vi "CRYStepSetup.vi"() -> ()   [LabVIEW 2013]
uses:
  CRYStepSetup Global.vi
panel:
  in  "StateOut":bool
  in  "Add Graph":bool
  in  "IconRing":u16(ring)
  in  "Add Graph Menu":bool
  in  "Control Visible":bool
  in  "Property":bool
  in  "TitleShowOnOff":bool
  in  "Save As":bool
  in  "Load":bool
  in  "Revert":bool
  out "SubVI Ref":refnum<vi>
  in  "stop":bool
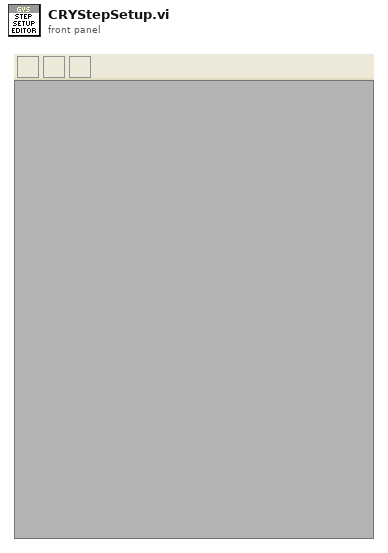
[diagram p1: front panel]
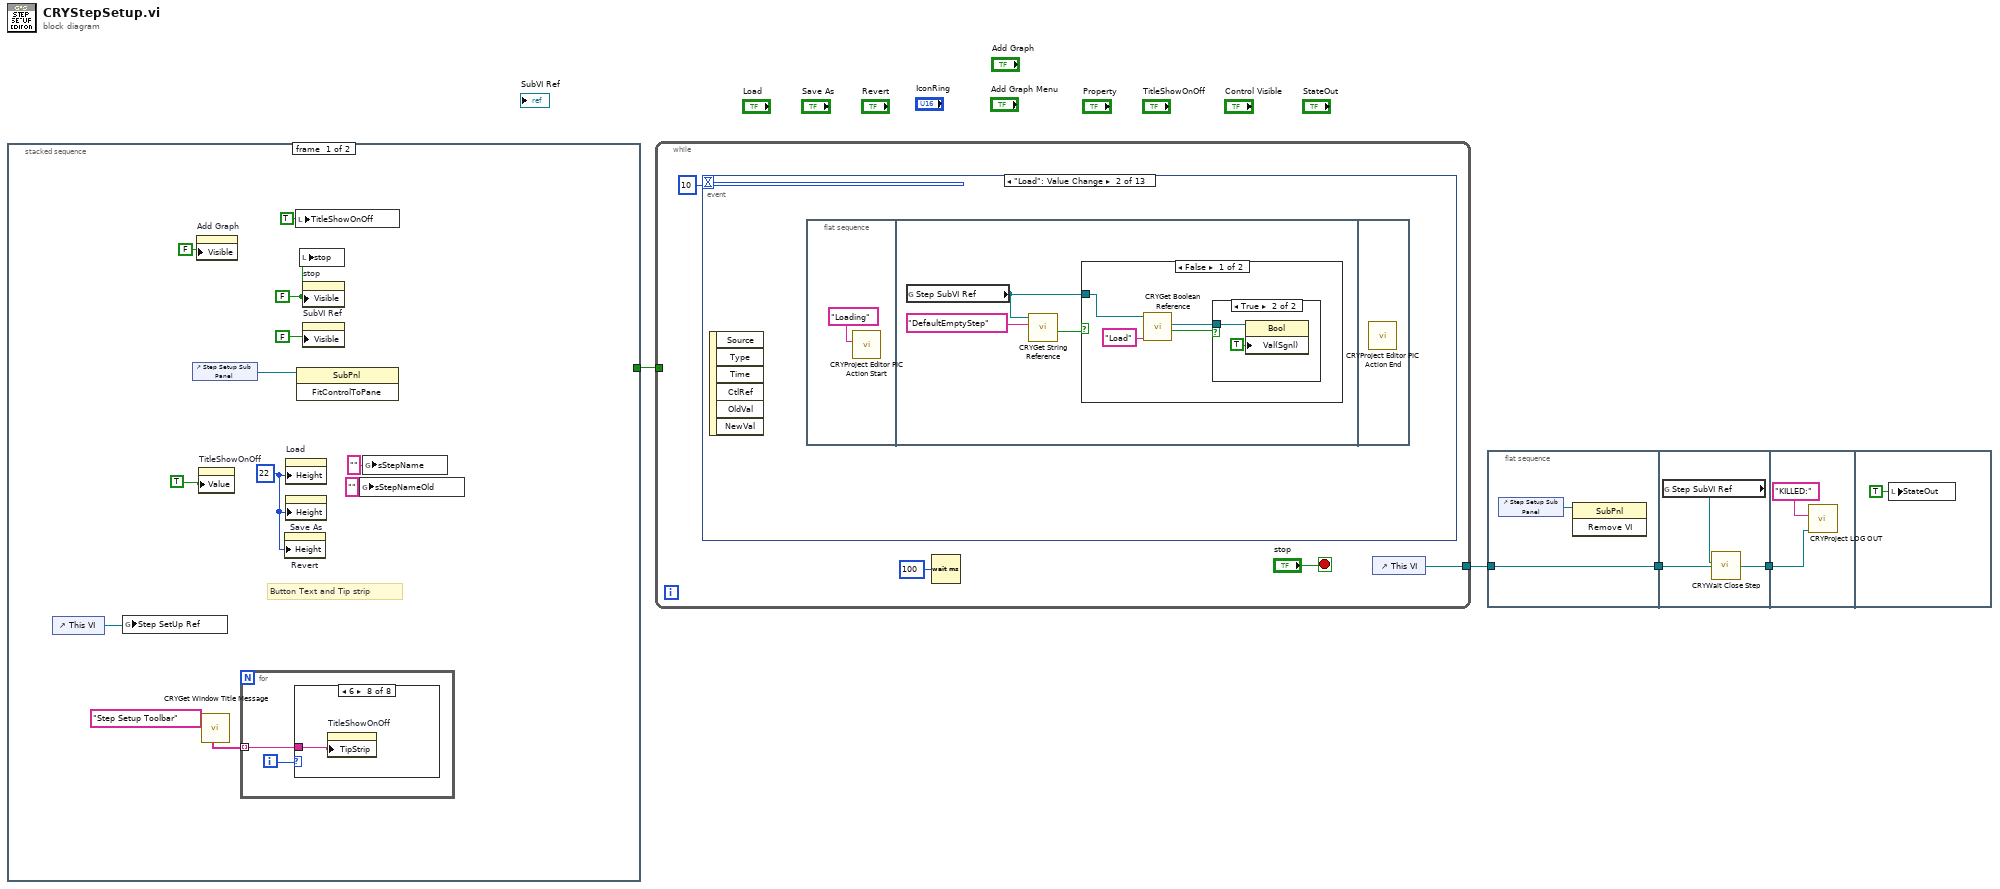
[diagram p0: block diagram]
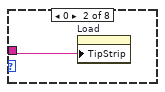
[diagram p3: hidden frame]
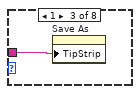
[diagram p4: hidden frame]
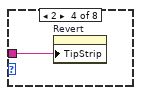
[diagram p5: hidden frame]
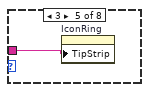
[diagram p6: hidden frame]
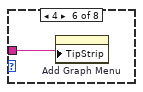
[diagram p7: hidden frame]
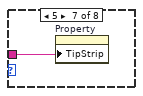
[diagram p8: hidden frame]
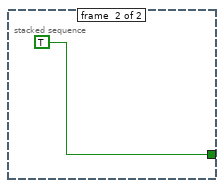
[diagram p9: hidden frame]
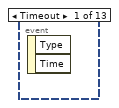
[diagram p10: hidden frame]
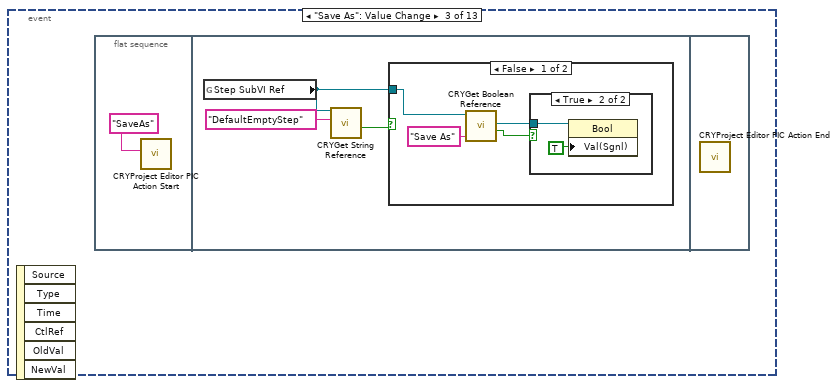
[diagram p13: hidden frame]
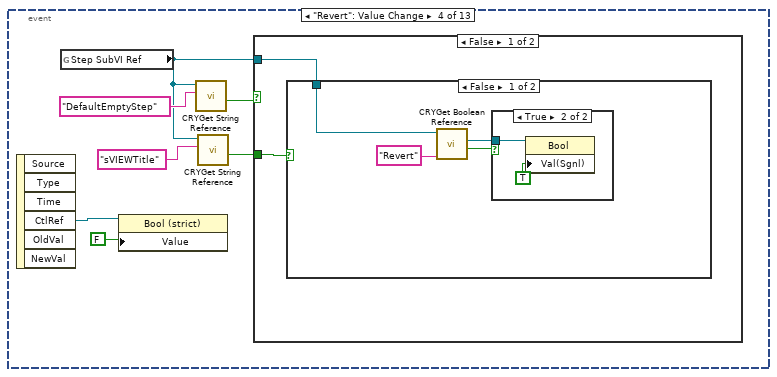
[diagram p16: hidden frame]
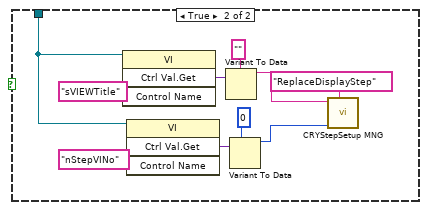
[diagram p18: hidden frame]
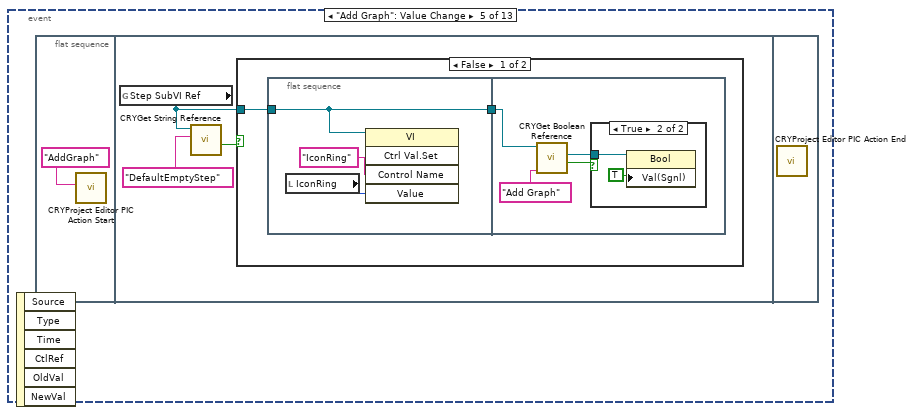
[diagram p20: hidden frame]
diagram:
  n1 = stacked-sequence {
    tunnel: [_ TRUE ("Step Setup Exist")] -> w4
    frame #0 {
      w15 = u32 22 ("Button Size:Height")
      w13 = FALSE ("Visible")
      # "Button Text and Tip strip"
      n2 = control-ref of="This VI"() -> (w5:refnum<vi>)
      n3 = global write "CRYStepSetup Global.vi" "Step SetUp Ref"(w5) -> ()
      n4 = control-ref of="Step Setup Sub Panel"() -> (w9:refnum<vi>)
      n5 = property on="Add Graph" class="Bool (strict)"("Visible"=FALSE) -> ()  [unwired: 2 in, 2 out]
      n6 = property on="TitleShowOnOff" class="Bool (strict)"("Value"=TRUE ("TitleShowOnOff")) -> ()  [unwired: 2 in, 2 out]
      n7 = call "CRYGet Window Title Message.vi"("Kind"="Step Setup Toolbar") -> ("Tip Strip"=w6:string[])  [unwired: 5 in, 5 out]
      n8 = for {
        tunnel: w6 -> [w17] mode=indexing
        i -> [w18]
        n9 = case shown="6" w18 {
          tunnel: w17 -> [_ w19 w20 w21 w22 w23 w24 w25]
          frame Default {
          }
          frame 0 {
            n10 = property on="Load" class="Bool (strict)"("TipStrip"=w19) -> ()  [unwired: 2 in, 2 out]
          }
          frame 1 {
            n11 = property on="Save As" class="Bool (strict)"("TipStrip"=w20) -> ()  [unwired: 2 in, 2 out]
          }
          frame 2 {
            n12 = property on="Revert" class="Bool (strict)"("TipStrip"=w21) -> ()  [unwired: 2 in, 2 out]
          }
          frame 3 {
            n13 = property on="IconRing" class="Ring (strict)"("TipStrip"=w22) -> ()  [unwired: 2 in, 2 out]
          }
          frame 4 {
            n14 = property on="Add Graph Menu" class="Bool (strict)"("TipStrip"=w23) -> ()  [unwired: 2 in, 2 out]
          }
          frame 5 {
            n15 = property on="Property" class="Bool (strict)"("TipStrip"=w24) -> ()  [unwired: 2 in, 2 out]
          }
          frame 6 {
            n16 = property on="TitleShowOnOff" class="Bool (strict)"("TipStrip"=w25) -> ()  [unwired: 2 in, 2 out]
          }
        }
      }
      n17 = property on="Revert" class="Bool (strict)"("Height"=w15) -> ()  [unwired: 2 in, 2 out]
      n18 = property on="Load" class="Bool (strict)"("Height"=w15) -> ()  [unwired: 2 in, 2 out]
      n19 = property on="Save As" class="Bool (strict)"("Height"=w15) -> ()  [unwired: 2 in, 2 out]
      n20 = local write "TitleShowOnOff"(TRUE ("TitleShowOnOff")) -> ()
      n21 = invoke class="SubPnl" method="FitControlToPane"(reference=w9) -> ()  [unwired: 2 in, 3 out]
      n22 = local write "stop"(w13) -> ()
      n23 = property on="stop" class="Bool (strict)"("Visible"=w13) -> ()  [unwired: 2 in, 2 out]
      n24 = property on="SubVI Ref" class="VIRef (strict)"("Visible"=FALSE) -> ()  [unwired: 2 in, 2 out]
      n25 = global write "CRYStepSetup Global.vi" "sStepNameOld"("" ("sStepName")) -> ()
      n26 = global write "CRYStepSetup Global.vi" "sStepName"("" ("sStepName")) -> ()
    }
    frame #1 {
    }
  }
  n27 = while {
    tunnel: w4 -> [_]
    tunnel: [w29] -> w3
    stop <- "stop" stop-if-true
    n28 = event shown="[1] \"Load\": Value Change" {
      selector: _ -> [_ _ _ _ _ _ _ _ _ _ _ _ _]
      dyn-events: _ -> [_ _ _ _ _ _ _ _ _ _ _ _ _]
      timeout: 10 -> [_ _ _ _ _ _ _ _ _ _ _ _ _]
      event Timeout {
        n29 = event-data() -> ()  [unwired: 3 out]
      }
      event "Load": Value Change {
        n30 = event-data() -> ()  [unwired: 7 out]
        n31 = flat-sequence {
          frame #0 {
            n32 = call "CRYProject Editor PIC Action Start.vi"("sData"="Loading" ("StateLabel")) -> ()  [unwired: 11 in]
          }
          frame #1 {
            n33 = global read "CRYStepSetup Global.vi" "Step SubVI Ref"() -> (w32:refnum<vi>)
            n34 = call "CRYGet String Reference.vi"("Label Name"="DefaultEmptyStep" ("element"), "VI Refnum"=w32) -> ("Find?"=w33:bool)  [unwired: 9 out]
            n35 = case shown="False" w33 {
              tunnel: w32 -> [w36 _]
              frame False {
                n36 = call "CRYGet Boolean Reference.vi"("Label Name"="Load", "VI Refnum"=w36) -> ("Exist?"=w35:bool, "Boolean Ref"=w38:refnum<vi>)  [unwired: 8 out]
                n37 = case shown="True" w35 {
                  tunnel: w38 -> [_ w40]
                  frame False {
                  }
                  frame True {
                    n38 = property class="Bool"(reference=w40, "Val(Sgnl)"=TRUE ("Value")) -> ()  [unwired: 1 in, 2 out]
                  }
                }
              }
              frame True {
              }
            }
          }
          frame #2 {
            n39 = call "CRYProject Editor PIC Action End.vi"() -> ()  [unwired: 12 in]
          }
        }
      }
      event "Save As": Value Change {
        n40 = event-data() -> ()  [unwired: 7 out]
        n41 = flat-sequence {
          frame #0 {
            n42 = call "CRYProject Editor PIC Action Start.vi"("sData"="SaveAs" ("StateLabel")) -> ()  [unwired: 11 in]
          }
          frame #1 {
            n43 = global read "CRYStepSetup Global.vi" "Step SubVI Ref"() -> (w42:refnum<vi>)
            n44 = call "CRYGet String Reference.vi"("Label Name"="DefaultEmptyStep" ("element"), "VI Refnum"=w42) -> ("Find?"=w43:bool)  [unwired: 9 out]
            n45 = case shown="False" w43 {
              tunnel: w42 -> [w46 _]
              frame False {
                n46 = call "CRYGet Boolean Reference.vi"("Label Name"="Save As" ("Label.Text"), "VI Refnum"=w46) -> ("Exist?"=w45:bool, "Boolean Ref"=w48:refnum<vi>)  [unwired: 8 out]
                n47 = case shown="True" w45 {
                  tunnel: w48 -> [_ w50]
                  frame False {
                  }
                  frame True {
                    n48 = property class="Bool"(reference=w50, "Val(Sgnl)"=TRUE ("Value")) -> ()  [unwired: 1 in, 2 out]
                  }
                }
              }
              frame True {
              }
            }
          }
          frame #2 {
            n49 = call "CRYProject Editor PIC Action End.vi"() -> ()  [unwired: 12 in]
          }
        }
      }
      event "Revert": Value Change {
        n50 = event-data() -> ("CtlRef"=w57:refnum<vi>)  [unwired: 6 out]
        n51 = global read "CRYStepSetup Global.vi" "Step SubVI Ref"() -> (w53:refnum<vi>)
        n52 = property class="Bool (strict)"(reference=w57, "Value"=FALSE) -> ()  [unwired: 1 in, 2 out]
        n53 = call "CRYGet String Reference.vi"("Label Name"="DefaultEmptyStep" ("element"), "VI Refnum"=w53) -> ("Find?"=w54:bool)  [unwired: 9 out]
        n54 = call "CRYGet String Reference.vi"("Label Name"="sVIEWTitle" ("Control Name"), "VI Refnum"=w53) -> ("Find?"=w51:bool)  [unwired: 9 out]
        n55 = case shown="False" w54 {
          tunnel: w53 -> [w59 _]
          tunnel: w51 -> [w58 _]
          frame False {
            n56 = case shown="False" w58 {
              tunnel: w59 -> [w61 w70]
              frame False {
                n57 = call "CRYGet Boolean Reference.vi"("Label Name"="Revert" ("Label.Text"), "VI Refnum"=w61) -> ("Exist?"=w60:bool, "Boolean Ref"=w63:refnum<vi>)  [unwired: 8 out]
                n58 = case shown="True" w60 {
                  tunnel: w63 -> [_ w65]
                  frame False {
                  }
                  frame True {
                    n59 = property class="Bool"(reference=w65, "Val(Sgnl)"=TRUE ("Value")) -> ()  [unwired: 1 in, 2 out]
                  }
                }
              }
              frame True {
                n60 = invoke class="VI" method="Ctrl Val.Get"(reference=w70, "Control Name"="sVIEWTitle") -> ("Get Control Value Variant"=w74:variant)  [unwired: 2 in, 3 out]
                n61 = invoke class="VI" method="Ctrl Val.Get"(reference=w70, "Control Name"="nStepVINo") -> ("Get Control Value Variant"=w71:variant)  [unwired: 2 in, 3 out]
                n62 = Variant To Data(type="", Variant=w74) -> (data=w73:string)  [unwired: 1 in, 1 out]
                n63 = Variant To Data(type=0, Variant=w71) -> (data=w69:i32)  [unwired: 1 in, 1 out]
                n64 = call "CRYStepSetup MNG.vi"("sAction"="ReplaceDisplayStep", "nData"=w69, "sData"=w73) -> ()  [unwired: 7 in, 2 out]
              }
            }
          }
          frame True {
          }
        }
      }
      event "Add Graph": Value Change {
        n65 = event-data() -> ()  [unwired: 7 out]
        n66 = flat-sequence {
          frame #0 {
            n67 = call "CRYProject Editor PIC Action Start.vi"("sData"="AddGraph" ("StateLabel")) -> ()  [unwired: 11 in]
          }
          frame #1 {
            n68 = global read "CRYStepSetup Global.vi" "Step SubVI Ref"() -> (w77:refnum<vi>)
            n69 = call "CRYGet String Reference.vi"("Label Name"="DefaultEmptyStep" ("element"), "VI Refnum"=w77) -> ("Find?"=w78:bool)  [unwired: 9 out]
            n70 = case shown="False" w78 {
              tunnel: w77 -> [w80 _]
              frame False {
                n71 = flat-sequence {
                  tunnel: [w84] -> w81
                  tunnel: w80 -> [w84]
                  tunnel: w81 -> [w86]
                  frame #0 {
                    n72 = local read "IconRing"() -> (w83:u16)
                    n73 = invoke class="VI" method="Ctrl Val.Set"(reference=w84, "Control Name"="IconRing", "Value"=w83) -> ()  [unwired: 2 in, 5 out]
                  }
                  frame #1 {
                    n74 = call "CRYGet Boolean Reference.vi"("Label Name"="Add Graph" ("Label.Text"), "VI Refnum"=w86) -> ("Exist?"=w85:bool, "Boolean Ref"=w88:refnum<vi>)  [unwired: 8 out]
                    n75 = case shown="True" w85 {
                      tunnel: w88 -> [_ w90]
                      frame False {
                      }
                      frame True {
                        n76 = property class="Bool"(reference=w90, "Val(Sgnl)"=TRUE ("Value")) -> ()  [unwired: 1 in, 2 out]
                      }
                    }
                  }
                }
              }
              frame True {
              }
            }
          }
          frame #2 {
            n77 = call "CRYProject Editor PIC Action End.vi"() -> ()  [unwired: 12 in]
          }
        }
      }
      event "IconRing": Mouse Down? {
        n78 = event-data() -> ()  [unwired: 9 out]
        n79 = flat-sequence {
          frame #0 {
            n80 = call "CRYProject Editor PIC Action Start.vi"("sData"="AddGraph" ("StateLabel")) -> ()  [unwired: 11 in]
          }
          frame #1 {
            n81 = property on="Add Graph" class="Bool (strict)"("Val(Sgnl)"=TRUE ("Value (Signaling)")) -> ()  [unwired: 2 in, 2 out]
          }
          frame #2 {
            n82 = call "CRYProject Editor PIC Action End.vi"() -> ()  [unwired: 12 in]
          }
        }
        n83 = event-data() -> ()  [unwired: 5 in, 1 out]
      }
      event "Add Graph Menu": Mouse Down? {
        n84 = event-data() -> ()  [unwired: 9 out]
        n85 = event-data("Button"=u16 2) -> ()  [unwired: 4 in, 1 out]
      }
      event "Add Graph Menu": Shortcut Menu Activation? {
        w96 = string[] ["Wave Graph", "XY Graph", "Polar", "Table", "Result", "Bar", "Text", "Digital", "Picture", "Intensity"]
        n86 = event-data() -> ("MenuRef"=w94:refnum<k9>)  [unwired: 7 out]
        n87 = Delete Menu Items(9:w94) -> (3:w95:refnum<k9>)  [unwired: 3 in, 1 out]
        n88 = Insert Menu Items(7:w96, 8:w96, 9:w95) -> ()  [unwired: 3 in, 3 out]
        n89 = event-data() -> ()  [unwired: 2 in, 1 out]
      }
      event "Add Graph Menu": Shortcut Menu Selection (User) {
        n90 = event-data() -> ("ItemTag"=w98:string)  [unwired: 8 out]
        n91 = flat-sequence {
          tunnel: [w99] -> _
          tunnel: "Below" ("ItemTag") -> [w103]
          tunnel: w98 -> [w99]
          frame #0 {
            n92 = case shown="\"Digital\"" w99 {
              tunnel: [0 1 2 3 4 5 6 7 8 8] -> w104
              frame "Wave Graph", Default {
              }
              frame "XY Graph" {
              }
              frame "Polar" {
              }
              frame "Table" {
              }
              frame "Result" {
              }
              frame "Bar" {
              }
              frame "Text" {
              }
              frame "Digital" {
              }
              frame "Picture" {
              }
              frame "Intensity" {
              }
            }
            n93 = case shown="\"Below\"" w103 {
              tunnel: ["ADD_WIN_L" "ADD_WIN_R" "ADD_WIN_A" "ADD_WIN_B"] -> w100
              frame "Left", Default {
              }
              frame "Right" {
              }
              frame "Above" {
              }
              frame "Below" {
              }
            }
            n94 = global read "CRYStepSetup Global.vi" "Step SubVI Ref"() -> (w102:refnum<vi>)
            n95 = local write "IconRing"(w104) -> ()
            n96 = invoke class="VI" method="Ctrl Val.Set"(reference=w102, "Control Name"="sAddGraphLRAB", "Value"=w100) -> ()  [unwired: 2 in, 5 out]
          }
          frame #1 {
            n97 = property on="Add Graph" class="Bool (strict)"("Val(Sgnl)"=TRUE ("Value (Signaling)")) -> ()  [unwired: 2 in, 2 out]
          }
        }
      }
      event "Add Graph Menu": Value Change {
        n98 = event-data() -> ("CtlRef"=w122:refnum<vi>)  [unwired: 6 out]
        n99 = property class="Bool (strict)"(reference=w122, "Value"=FALSE) -> ()  [unwired: 1 in, 2 out]
        n100 = global read "CRYStepSetup Global.vi" "Step SubVI Ref"() -> (w120:refnum<vi>)
        n101 = call "CRYGet String Reference.vi"("Label Name"="DefaultEmptyStep" ("element"), "VI Refnum"=w120) -> ("Find?"=w123:bool)  [unwired: 9 out]
        n102 = case shown="False" w123 {
          tunnel: w120 -> [w125 _]
          frame False {
            n103 = call "CRYGet Boolean Reference.vi"("Label Name"="Add Graph Menu" ("Label.Text"), "VI Refnum"=w125) -> ("Boolean Ref"=w128:refnum<vi>)  [unwired: 9 out]
            n104 = property class="Bool"(reference=w128, "Val(Sgnl)"=TRUE ("Value")) -> ()  [unwired: 1 in, 2 out]
          }
          frame True {
          }
        }
      }
      event "Property": Value Change {
        n105 = event-data() -> ()  [unwired: 7 out]
        n106 = flat-sequence {
          frame #0 {
            n107 = call "CRYProject Editor PIC Action Start.vi"("sData"="Property" ("StateLabel")) -> ()  [unwired: 11 in]
          }
          frame #1 {
            n108 = global read "CRYStepSetup Global.vi" "Step SubVI Ref"() -> (w130:refnum<vi>)
            n109 = call "CRYGet String Reference.vi"("Label Name"="DefaultEmptyStep" ("element"), "VI Refnum"=w130) -> ("Find?"=w131:bool)  [unwired: 9 out]
            n110 = case shown="False" w131 {
              tunnel: w130 -> [w133 _]
              frame False {
                n111 = call "CRYGet Boolean Reference.vi"("Label Name"="Property" ("Label.Text"), "VI Refnum"=w133) -> ("Boolean Ref"=w136:refnum<vi>)  [unwired: 9 out]
                n112 = property class="Bool"(reference=w136, "Val(Sgnl)"=TRUE ("Value")) -> ()  [unwired: 1 in, 2 out]
              }
              frame True {
              }
            }
          }
          frame #2 {
            n113 = call "CRYProject Editor PIC Action End.vi"() -> ()  [unwired: 12 in]
          }
        }
      }
      event "TitleShowOnOff": Value Change {
        n114 = event-data() -> ("NewVal"=w138:bool)  [unwired: 6 out]
        n115 = flat-sequence {
          tunnel: w138 -> [w140]
          tunnel: [w140] -> w137
          tunnel: w137 -> [w142]
          frame #0 {
            n116 = call "CRYProject Editor PIC Action Start.vi"("sData"="TitleShowOnOff" ("StateLabel")) -> ()  [unwired: 11 in]
          }
          frame #1 {
            n117 = global read "CRYStepSetup Global.vi" "Step SubVI Ref"() -> (w141:refnum<vi>)
            n118 = call "CRYGet String Reference.vi"("Label Name"="DefaultEmptyStep" ("element"), "VI Refnum"=w141) -> ("Find?"=w143:bool)  [unwired: 9 out]
            n119 = case shown="False" w143 {
              tunnel: w142 -> [w147 _]
              tunnel: w141 -> [w146 _]
              frame False {
                n120 = call "CRYGet Boolean Reference.vi"("Label Name"="TitleShowOnOff" ("Label.Text"), "VI Refnum"=w146) -> ("Exist?"=w145:bool, "Boolean Ref"=w149:refnum<vi>)  [unwired: 8 out]
                n121 = case shown="True" w145 {
                  tunnel: w149 -> [_ w151]
                  tunnel: w147 -> [_ w150]
                  frame False {
                  }
                  frame True {
                    n122 = property class="Bool"(reference=w151, "Val(Sgnl)"=w150) -> ()  [unwired: 1 in, 2 out]
                  }
                }
              }
              frame True {
              }
            }
          }
          frame #2 {
            n123 = call "CRYProject Editor PIC Action End.vi"() -> ()  [unwired: 12 in]
          }
        }
      }
      event "Control Visible": Value Change {
        n124 = event-data() -> ("NewVal"=w152:bool)  [unwired: 6 out]
        n125 = property on="Property" class="Bool (strict)"("Visible"=w152) -> ()  [unwired: 2 in, 2 out]
        n126 = property on="TitleShowOnOff" class="Bool (strict)"("Visible"=w152) -> ()  [unwired: 2 in, 2 out]
        n127 = property on="Add Graph Menu" class="Bool (strict)"("Visible"=w152) -> ()  [unwired: 2 in, 2 out]
        n128 = property on="IconRing" class="Ring (strict)"("Visible"=w152) -> ()  [unwired: 2 in, 2 out]
      }
    }
    n129 = Wait (ms)(milliseconds to wait=u32 100) -> ()  [unwired: 1 out]
    n130 = control-ref of="This VI"() -> (w29:refnum<vi>)
  }
  n131 = flat-sequence {
    tunnel: w3 -> [w153]
    tunnel: [w153] -> w2
    tunnel: w2 -> [w156]
    tunnel: [w156] -> w1
    tunnel: w1 -> [w157]
    frame #0 {
      n132 = control-ref of="Step Setup Sub Panel"() -> (w154:refnum<vi>)
      n133 = invoke class="SubPnl" method="Remove VI"(reference=w154) -> ()  [unwired: 2 in, 3 out]
    }
    frame #1 {
      n134 = global read "CRYStepSetup Global.vi" "Step SubVI Ref"() -> (w155:refnum<vi>)
      n135 = call "CRYWait Close Step.vi"("vi reference"=w155) -> ()  [unwired: 11 in]
    }
    frame #2 {
      n136 = call "CRYProject LOG OUT.vi"("pVIRef"=w157, "sData"="KILLED:") -> ()  [unwired: 10 in]
    }
    frame #3 {
      n137 = local write "StateOut"(TRUE ("StateOut")) -> ()
    }
  }
